vi "PicoScope2000Settings.vi"(1 "Unit Info":T1, 4 "Channel B Settings":T2 {"Range" items=["20 mV", "50 mV", "100 mV", "200 mV", "500 mV", "1 V", "2 V", "5 V", "10 V", "20 V"]; "Coupling" items=["AC", "DC"]}, 5 "Channel A Settings":T2 {"Range" items=["20 mV", "50 mV", "100 mV", "200 mV", "500 mV", "1 V", "2 V", "5 V", "10 V", "20 V"]; "Coupling" items=["AC", "DC"]}, 6 "Trigger Settings":T3 {"Trigger Direction" items=["Rising", "Falling"]; "Trigger Threshold (V)" format="%.3f"}, 7 "Max ADC value":i16, 8 "handle in":i16, 9 "error in":errorcluster) -> (0 "Enabled Array":i16[](array[numeric]), 2 "handle out":i16, 3 "error out":errorcluster)   [LabVIEW 2009]
doc: "This VI is used to set up the oscilloscope. The inputs are clusters for setting channel and simple trigger settings. Advanced triggers can be set up using PicoScope3000aAdvancedTriggerSettings.vi"
uses:
  ps2000.dll
  PicoScope2000AnalogChannelSettings.ctl
panel:
  in  "Channel D range":i16
  in  "Channel D dc":i16
  in  "Channel D enabled":i16
  in  "Channel C range":i16
  in  "Channel C dc":i16
  in  "Channel C enabled":i16
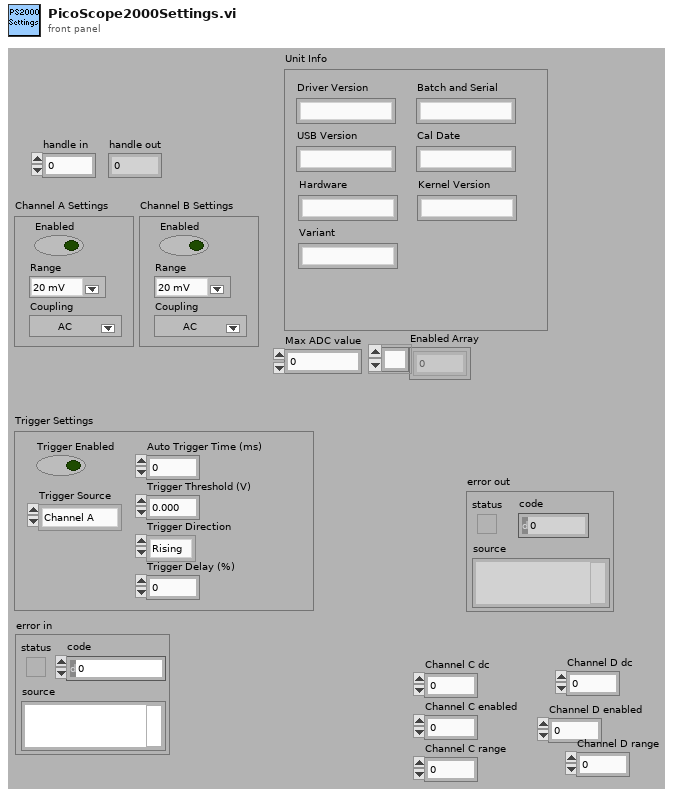
[diagram p1: front panel]
types:
  T1 = cluster{"Driver Version":string, "USB Version":string, "Hardware":string, "Variant":string, "Batch and Serial":string, "Cal Date":string, "Kernel Version":string}
  T2 = typedef "PicoScope2000AnalogChannelSettings.ctl" = cluster{"Enabled":bool, "Coupling":i16, "Range":u16}
  T3 = cluster{"Trigger Enabled":bool, "Trigger Source":enum16{"Channel A", "Channel B"}, "Trigger Threshold (V)":dbl, "Trigger Direction":i16, "Trigger Delay (%)":i16, "Auto Trigger Time (ms)":i16}
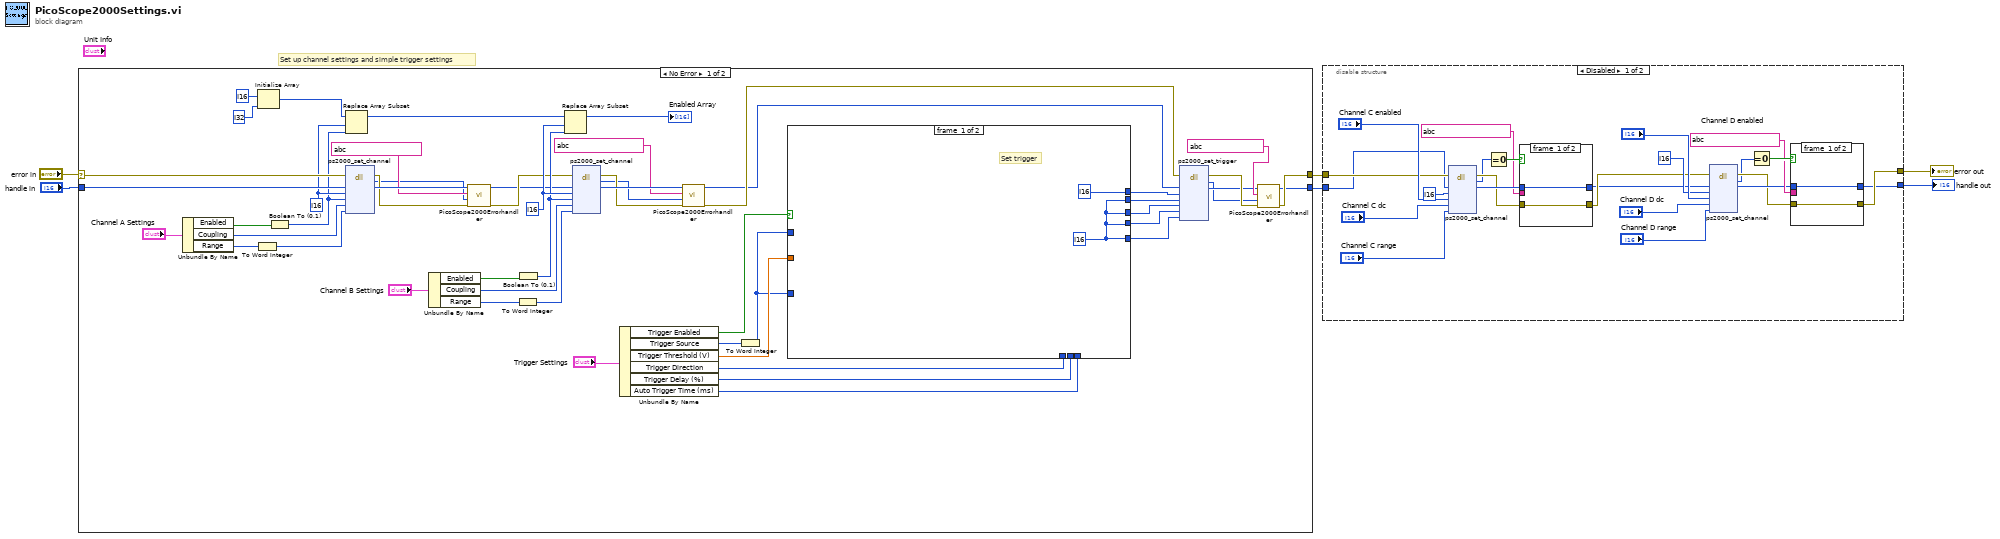
[diagram p0: block diagram]
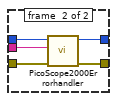
[diagram p2: hidden frame]
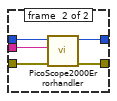
[diagram p3: hidden frame]
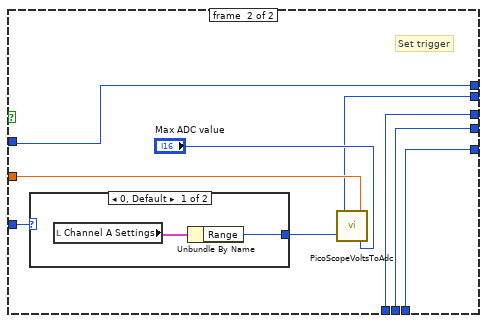
[diagram p5: hidden frame]
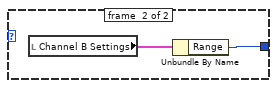
[diagram p6: hidden frame]
diagram:
  # "Set up channel settings and simple trigger settings"
  n1 = case shown="No Error" "error in" {
    selector: "error in" -> [w55 w75]
    tunnel: "handle in" -> [w54 w74]
    tunnel: [w17 w74] -> w3
    tunnel: [w18 w75] -> w4
    frame #0 {
      w32 = i16 ? ("channel")
      w35 = i16 ? ("channel")
      n2 = Unbundle By Name("Channel A Settings") -> ("Enabled"=w53:bool, "Coupling"=w52:i16, "Range"=w51:u16)
      n3 = To Word Integer(number=w51) -> (16bit integer=w40:i16)
      n4 = Initialize Array(i16 ? ("element"), i32 ? ("dimension size")) -> (w36:i16[])
      n5 = Boolean To (0,1)(Boolean=w53) -> (0, 1=w34:i16)
      n6 = Replace Array Subset(array=w36, new element=w34, index=w35) -> (w33:i16[])
      n7 = dll-call lib="PS2000.dll" fn="ps2000_set_channel"(error in=w55, "handle"=w54, "channel"=w35, "enabled"=w34, "dc"=w52, "range"=w40) -> (error out=w28:errorcluster, "return"=w16:i16, "handle"=w29:i16)  [unwired: 6 in, 1 out]
      n8 = Unbundle By Name("Channel B Settings") -> ("Enabled"=w50:bool, "Coupling"=w49:i16, "Range"=w41:u16)
      n9 = call "PicoScope2000Errorhandler.vi"("Handle in"=w29, "API function"=string ? ("source"), "Return"=w16, "error in (no error)"=w28) -> ("Handle out"=w26:i16, "error out"=w27:errorcluster)  [unwired: 5 in]
      n10 = To Word Integer(number=w41) -> (16bit integer=w39:i16)
      n11 = Boolean To (0,1)(Boolean=w50) -> (0, 1=w31:i16)
      n12 = Replace Array Subset(array=w33, new element=w31, index=w32) -> (→"Enabled Array":i16[])
      n13 = dll-call lib="PS2000.dll" fn="ps2000_set_channel"(error in=w27, "handle"=w26, "channel"=w32, "enabled"=w31, "dc"=w49, "range"=w39) -> (error out=w20:errorcluster, "return"=w15:i16, "handle"=w24:i16)  [unwired: 6 in, 1 out]
      n14 = Unbundle By Name("Trigger Settings") -> ("Trigger Enabled"=w48:bool, "Trigger Source"=w43:enum16{"Channel A", "Channel B"}, "Trigger Threshold (V)"=w44:dbl, "Trigger Direction"=w47:i16, "Trigger Delay (%)"=w46:i16, "Auto Trigger Time (ms)"=w45:i16)
      n15 = call "PicoScope2000Errorhandler.vi"("Handle in"=w24, "API function"=string ? ("source"), "Return"=w15, "error in (no error)"=w20) -> ("Handle out"=w22:i16, "error out"=w23:errorcluster)  [unwired: 5 in]
      n16 = To Word Integer(number=w43) -> (16bit integer=w42:i16)
      n17 = case shown="True" w48 {
        tunnel: w42 -> [_ w61]
        tunnel: w47 -> [_ w63]
        tunnel: w46 -> [_ w64]
        tunnel: w45 -> [_ w65]
        tunnel: w44 -> [_ w67]
        tunnel: w42 -> [_ w69]
        tunnel: [i16 ? ("source") w61] -> w14
        tunnel: [w59 w65] -> w13
        tunnel: [w59 w64] -> w12
        tunnel: [w59 w63] -> w11
        tunnel: [w59 w62] -> w10
        frame #0 {
          w59 = i16 ? ("auto_trigger_ms")
          # "Set trigger"
        }
        frame #1 {
          # "Set trigger"
          n18 = case shown="0, Default" w69 {
            tunnel: [w70 w72] -> w68
            frame #0 {
              n19 = local read "Channel A Settings"() -> (w71:T2)
              n20 = Unbundle By Name(w71) -> ("Range"=w70:u16)
            }
            frame #1 {
              n21 = local read "Channel B Settings"() -> (w73:T2)
              n22 = Unbundle By Name(w73) -> ("Range"=w72:u16)
            }
          }
          n23 = call "PicoScopeVoltsToAdc.vi"("Max_adc"="Max ADC value", "Units"=w67, "Range Index"=w68) -> ("ADC count"=w62:i16)
        }
      }
      n24 = dll-call lib="ps2000.dll" fn="ps2000_set_trigger"(error in=w23, "handle"=w22, "source"=w14, "threshold"=w10, "direction"=w11, "delay"=w12, "auto_trigger_ms"=w13) -> (error out=w9:errorcluster, "return"=w7:i16, "handle"=w8:i16)  [unwired: 7 in, 1 out]
      n25 = call "PicoScope2000Errorhandler.vi"("Handle in"=w8, "API function"=string ? ("source"), "Return"=w7, "error in (no error)"=w9) -> ("Handle out"=w17:i16, "error out"=w18:errorcluster)  [unwired: 5 in]
    }
    frame #1 {
    }
  }
  n26 = disable-structure shown="Disabled" {
    disable-tunnel: w4 -> [w95 w115]
    disable-tunnel: w3 -> [w94 w114]
    disable-tunnel: [w77 w115] -> w2
    disable-tunnel: [w76 w114] -> w1
    frame #0 {
      n27 = dll-call lib="PS2000.dll" fn="ps2000_set_channel" label="ps2000_set_channel_C"(error in=w95, "handle"=w94, "channel"=i16 ?, "enabled"="Channel C enabled", "dc"="Channel C dc", "range"="Channel C range") -> (error out=w86:errorcluster, "return type"=w85:i16, "handle"=w88:i16)  [unwired: 6 in, 1 out]
      n28 = Equal To 0?(x=w85) -> (x = 0?=w89:bool)
      n29 = case shown="True" w89 {
        tunnel: [w107 w113] -> w84
        tunnel: w86 -> [w107 w112]
        tunnel: string ? ("source") -> [_ w111]
        tunnel: w88 -> [w108 w110]
        tunnel: [w108 w109] -> w83
        frame #0 {
        }
        frame #1 {
          n30 = call "PicoScope2000Errorhandler.vi"("Handle in"=w110, "API function"=w111, "error in (no error)"=w112) -> ("Handle out"=w109:i16, "error out"=w113:errorcluster)  [unwired: 6 in]
        }
      }
      n31 = dll-call lib="PS2000.dll" fn="ps2000_set_channel"(error in=w84, "handle"=w83, "channel"=i16 ?, "enabled"="Channel D enabled", "dc"="Channel D dc", "range"="Channel D range") -> (error out=w79:errorcluster, "return type"=w78:i16, "handle"=w80:i16)  [unwired: 6 in, 1 out]
      n32 = Equal To 0?(x=w78) -> (x = 0?=w82:bool)
      n33 = case shown="True" w82 {
        tunnel: [w100 w106] -> w77
        tunnel: w79 -> [w100 w105]
        tunnel: string ? ("source") -> [_ w104]
        tunnel: w80 -> [w101 w103]
        tunnel: [w101 w102] -> w76
        frame #0 {
        }
        frame #1 {
          n34 = call "PicoScope2000Errorhandler.vi"("Handle in"=w103, "API function"=w104, "error in (no error)"=w105) -> ("Handle out"=w102:i16, "error out"=w106:errorcluster)  [unwired: 6 in]
        }
      }
    }
    frame #1 {
    }
  }
  "handle out" <- w1
  "error out" <- w2
